vi "Read PNG.vi"() -> ()   [LabVIEW 2021, in "Renderer Tests.lvclass"]
uses:
  Renderer Tests.lvclass
  Renderer Tests.lvclass/Renderer Tests.ctl
  <vilib>/picture/picture.llb/Draw True-Color Pixmap.vi
panel:
  out "size(s)":i32
  out "24-bit pixmap":u32[][](array[numeric]) format="%x"
  out "2D Picture 2":picture
  out "2D Picture":picture
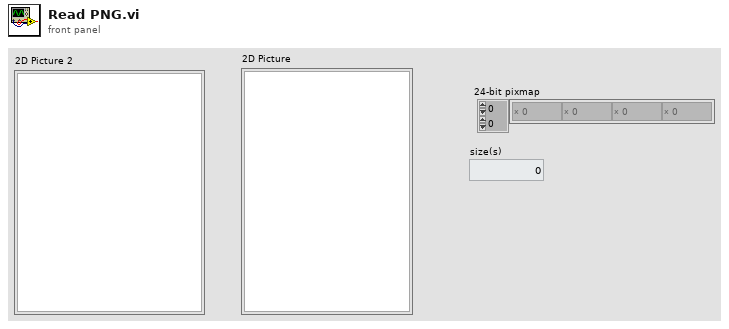
[diagram p1: front panel]
types:
  T1 = cluster{"left":i16, "top":i16, "right":i16, "bottom":i16}
  T2 = typedef "imagedata.ctl" = cluster{"image type":i32, "image depth":i32, "image":u8[], "mask":u8[], "colors":u32[], "Rectangle":cluster{"left":i16, "top":i16, "right":i16, "bottom":i16}}
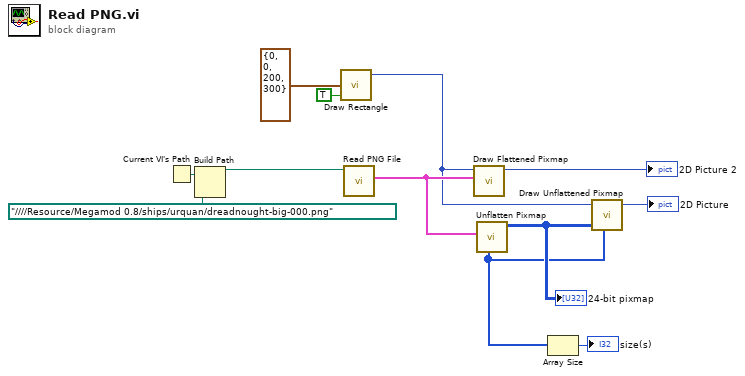
[diagram p0: block diagram]
diagram:
  n1 = Current VI's Path() -> (path=w12:path)
  n2 = Build Path(base path=w12, name or relative path=path "../../../../Resource/Megamod 0.8/ships/urquan/dreadnought-big-000.png" ("Path")) -> (appended path=w11:path)
  n3 = call <vilib>:"Draw Rectangle.vi"("rect"=T1 {"left"=0, "top"=0, "right"=200, "bottom"=300}, "fill?(F)"=TRUE) -> ("new picture"=w4:picture)  [unwired: 7 in]
  n4 = call <vilib>:"Read PNG File.vi"("path to PNG file"=w11) -> ("image data"=w7:T2)  [unwired: 8 in, 2 out]
  n5 = call <vilib>:"Draw Flattened Pixmap.vi"("image data"=w7, "picture"=w4) -> ("new picture"=→"2D Picture 2":picture)  [unwired: 7 in]
  n6 = call <vilib>:"Unflatten Pixmap.vi"("image data"=w7) -> ("24-bit pixmap"=w3:u32[][], "mask"=w2:u8[])  [unwired: 4 in, 5 out]
  "24-bit pixmap" <- w3
  n7 = Array Size(array=w2) -> (size(s)=→"size(s)":i32)
  n8 = call-poly <vilib>:"Draw Unflattened Pixmap.vi"("picture"=w4, "data (RGB format)"=w3, "mask"=w2) -> ("new picture"=→"2D Picture":picture)  [unwired: 6 in]
